vi "Read Attributes.vi"(11 "Display Game Board Msg":refnum<class "Display Game Board Msg.lvclass">) -> (2 "Payload":T1)   [LabVIEW 2017, in "Screen Interface.lvlib" / "Display Game Board Msg.lvclass"]
uses:
  Display Game Board Msg.lvclass
  Display Game Board Msg.lvclass/Display Game Board Msg.ctl
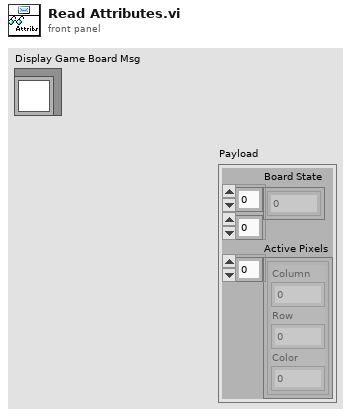
[diagram p1: front panel]
types:
  T1 = cluster{"Board State":u32[][], "Active Pixels":cluster{"Column":u8, "Row":u8, "Color":u32}[]}
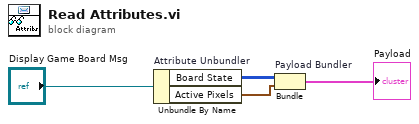
[diagram p0: block diagram]
diagram:
  n1 = Unbundle By Name "Attribute Unbundler"("Display Game Board Msg") -> ("Board State"=w2:u32[][], "Active Pixels"=w1:cluster{"Column":u8, "Row":u8, "Color":u32}[])
  n2 = Bundle "Payload Bundler"("Board State"=w2, "Active Pixels"=w1) -> (→"Payload":T1)  [unwired: 1 in]
